vi "AutoMap Channels.vi"(8 "error in (no error)":errorcluster, 10 "Write Channels":string[](array[string]), 11 "Read Channels":string[](array[string])) -> (0 "error out":errorcluster, 3 "Settings":T1)   [LabVIEW 2024]
uses:
  <userlib>/SimpleSysDef/_SubVIs/Add System Mappings_Settings_Channel Pairs.ctl
  <userlib>/SimpleSysDef/Simple SysDef API.lvlib
  NationalInstruments.VeriStand
  <userlib>/SimpleSysDef/_SubVIs/Add System Mappings_Settings.ctl
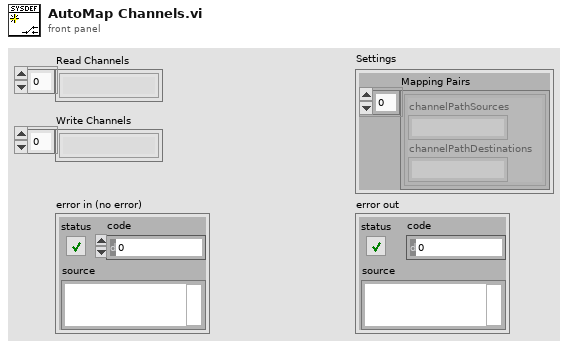
[diagram p1: front panel]
types:
  T1 = typedef "Simple SysDef API.lvlib/Add System Mappings_Settings.ctl" = cluster{"Mapping Pairs":T2[]}
  T2 = typedef "Simple SysDef API.lvlib/Add System Mappings_Settings_Channel Pairs.ctl" = cluster{"channelPathSources":string, "channelPathDestinations":string}
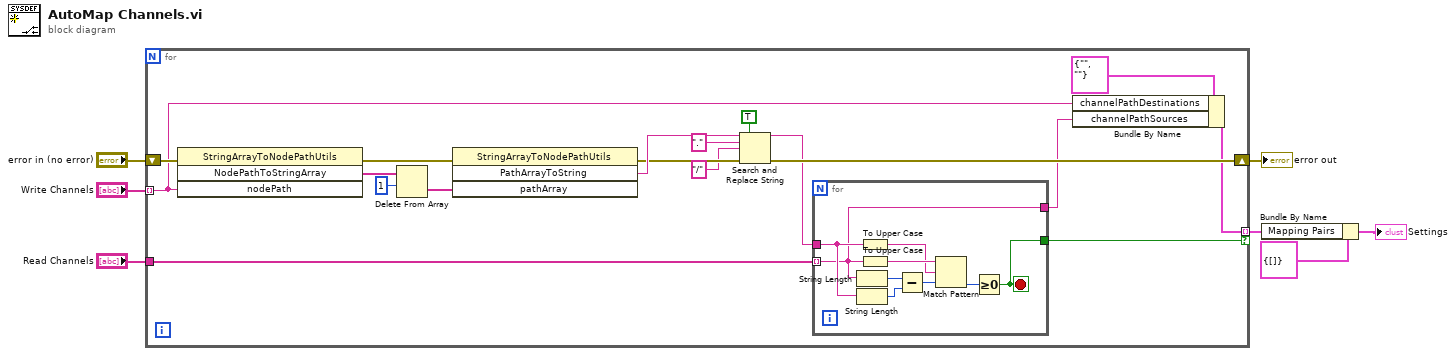
[diagram p0: block diagram]
diagram:
  n1 = for {
    tunnel: "Write Channels" -> [w9] mode=indexing
    shift-right: [w18] -> w4
    shift-left: "error in (no error)" -> [w21]
    tunnel: "Read Channels" -> [w14]
    tunnel: [w10] -> w2 mode=indexing if=w12
    n2 = invoke class="StringArrayToNodePathUtils" method="NodePathToStringArray"(error in=w21, "nodePath"=w9) -> (error out=w23:errorcluster, "NodePathToStringArray"=w25:string[])  [unwired: 2 in, 2 out]
    n3 = Delete From Array(array=w25, length=1) -> (deleted portion=w22:string[])  [unwired: 1 in, 1 out]
    n4 = invoke class="StringArrayToNodePathUtils" method="PathArrayToString"(error in=w23, "pathArray"=w22) -> (error out=w19:errorcluster, "PathArrayToString"=w20:string)  [unwired: 2 in, 2 out]
    n5 = Search and Replace String(replace all?=TRUE ("replace all? (F)"), input string=w20, search string=".", replace string="/" ("replace string (\"\")"), error in=w19) -> (result string=w13:string, error out=w18:errorcluster)  [unwired: 3 in, 2 out]
    n6 = for {
      tunnel: w14 -> [w27] mode=indexing
      tunnel: w13 -> [w32]
      tunnel: [w27] -> w8
      tunnel: [w26] -> w12
      stop <- w26 stop-if-true
      n7 = String Length(string=w27) -> (length=w31:i32)
      n8 = String Length(string=w32) -> (length=w30:i32)
      n9 = To Upper Case(1:w32) -> (0:w33:string)
      n10 = To Upper Case(1:w27) -> (0:w34:string)
      n11 = Subtract(x=w31, y=w30) -> (x-y=w29:i32)
      n12 = Match Pattern(string=w34, regular expression=w33, offset (0)=w29) -> (offset past match=w28:i32)  [unwired: 3 out]
      n13 = Greater Or Equal To 0?(x=w28) -> (x >= 0?=w26:bool)
    }
    n14 = Bundle By Name(cluster=T2 {"channelPathSources"="", "channelPathDestinations"=""} ("Mapping Pairs"), "channelPathDestinations"=w9, "channelPathSources"=w8) -> (w10:T2)
  }
  "error out" <- w4
  n15 = Bundle By Name(cluster=T1 {"Mapping Pairs"=[]} ("Settings"), "Mapping Pairs"=w2) -> (→"Settings":T1)
